vi "YKMW100 Measurement Single Analog Channel Data.vi"(0 "VISA session":refnum<visa-resource-name>, 1 "How to Get Data (F:Binary)":bool, 5 "Start Channel (001)":string="001", 9 "End Channel (001)":string="001", 11 "error in (no error)":errorcluster, 12 "Decimal Place List (no array)":i8[](array[numeric]) min=-1 max=4 step=1) -> (2 "Date Time":T1={"Year"=0, "Month"=1, "Day"=1, "Hour"=0, "Minute"=0, "Second"=0} {"Second" max=59 step=1; "Minute" max=59 step=1; "Hour" max=23 step=1; "Day" min=1 max=31 step=1; "Month" min=1 max=12 step=1; "Year" max=99 step=1}, 4 "dup VISA session":refnum<visa-resource-name>, 6 "Channel List":string[](array[string]), 8 "Data List":dbl[](array[numeric]) format="%.4f", 10 "Data Status List":T3(array[ring]), 13 "Alarm Status List":T2(array[cluster]), 14 "Decimal Place List":i8[](array[numeric]) min=-1 max=4 step=1, 15 "error out":errorcluster)   [LabVIEW 2009]
doc: "This VI gets the measurement data by ASCII or BINARY.\nWhen the data is formated by binary and the decimal place list is no array, this VI gets the unit and decimal point information by YKMW100 Unit Decimal Point.vi."
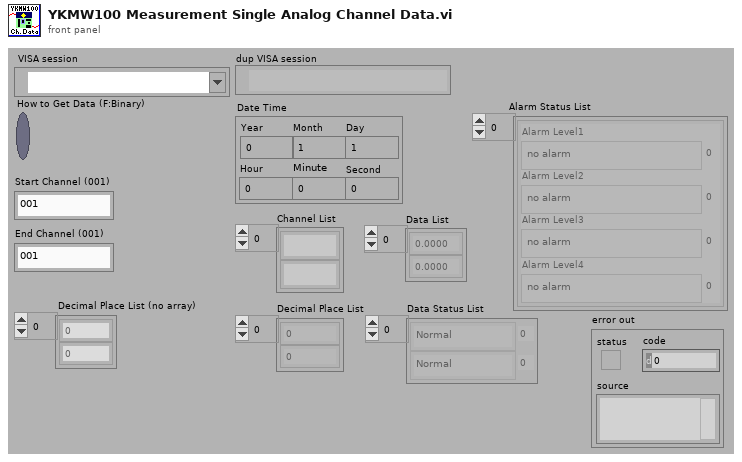
[diagram p1: front panel]
types:
  T1 = cluster{"Year":u8, "Month":u8, "Day":u8, "Hour":u8, "Minute":u8, "Second":u8}
  T2 = cluster{"Alarm Level1":enum8{"no alarm", "H (upper limit)", "L (lower Limit)", "h (defference upper limit)", "l (difference lower limit)", "R (upper limit on rate of change)", "r (lower limit on rate of change)"}, "Alarm Level2":enum8{"no alarm", "H (upper limit)", "L (lower Limit)", "h (defference upper limit)", "l (difference lower limit)", "R (upper limit on rate of change)", "r (lower limit on rate of change)"}, "Alarm Level3":enum8{"no alarm", "H (upper limit)", "L (lower Limit)", "h (defference upper limit)", "l (difference lower limit)", "R (upper limit on rate of change)", "r (lower limit on rate of change)"}, "Alarm Level4":enum8{"no alarm", "H (upper limit)", "L (lower Limit)", "h (defference upper limit)", "l (difference lower limit)", "R (upper limit on rate of change)", "r (lower limit on rate of change)"}}[]
  T3 = enum8{"Normal", "Differential Input", "Skip", "Over", "Error"}[]
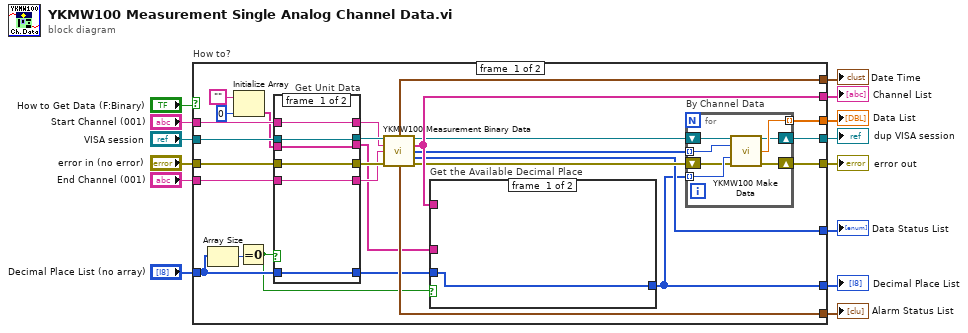
[diagram p0: block diagram]
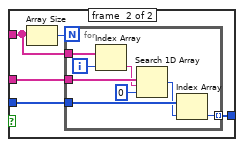
[diagram p2: hidden frame]
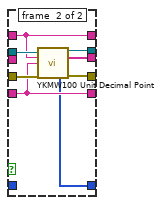
[diagram p3: hidden frame]
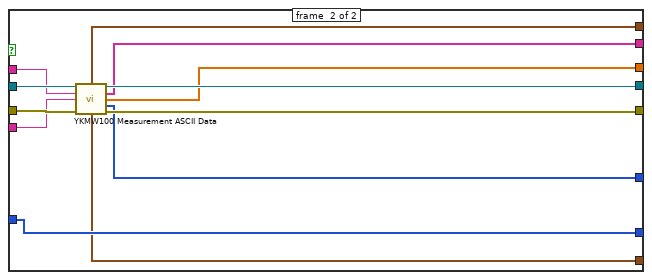
[diagram p4: hidden frame]
diagram:
  n1 = case "How to?" shown="False" "How to Get Data (F:Binary)" {
    tunnel: "VISA session" -> [w41 w87]
    tunnel: "error in (no error)" -> [w40 w86]
    tunnel: [w31 w82] -> w12
    tunnel: [w30 w81] -> w11
    tunnel: "End Channel (001)" -> [w38 w85]
    tunnel: "Start Channel (001)" -> [w39 w84]
    tunnel: "Decimal Place List (no array)" -> [w37 w88]
    tunnel: [w15 w88] -> w8
    tunnel: [w28 w83] -> w7
    tunnel: [w29 w78] -> w6
    tunnel: [w16 w79] -> w5
    tunnel: [w27 w80] -> w4
    tunnel: [w26 w77] -> w1
    frame #0 {
      n2 = Array Size(array=w37) -> (size(s)=w36:i32)
      n3 = Initialize Array("", 0) -> (w20:string[])
      n4 = Equal To 0?(x=w36) -> (x = 0?=w23:bool)
      n5 = case "Get Unit Data" shown="True" w23 {
        tunnel: w41 -> [w68 w76]
        tunnel: w40 -> [w67 w75]
        tunnel: w39 -> [w66 w72]
        tunnel: w38 -> [w65 w71]
        tunnel: [w67 w74] -> w34
        tunnel: [w68 w73] -> w35
        tunnel: [w66 w72] -> w33
        tunnel: [w65 w71] -> w32
        tunnel: [w64 w70] -> w24
        tunnel: w37 -> [w64 _]
        tunnel: [w63 w69] -> w25
        tunnel: w20 -> [w63 _]
        frame #0 {
        }
        frame #1 {
          n6 = call <instrlib>:"YKMW100 Unit Decimal Point.vi"("VISA session"=w76, "Start Channel (001)"=w72, "End Channel (001)"=w71, "error in (no error)"=w75) -> ("dup VISA session"=w73:refnum<visa-resource-name>, "Channel List"=w69:string[], "Decimal Place List"=w70:i8[], "error out"=w74:errorcluster)  [unwired: 6 in, 2 out]
        }
      }
      n7 = call <instrlib>:"YKMW100 Measurement Binary Data.vi"("VISA session"=w35, "Start Channel (001)"=w33, "End Channel (001)"=w32, "error in (no error)"=w34) -> ("Date Time"=w28:T1, "dup VISA session"=w19:refnum<visa-resource-name>, "Channel List"=w26:string[], "Data List"=w18:i32[], "Data Status List"=w16:T3, "Alarm Status List"=w27:T2, "error out"=w17:errorcluster)  [unwired: 5 in]
      n8 = case "Get the Available Decimal Place" shown="True" w23 {
        tunnel: w25 -> [_ w47]
        tunnel: w24 -> [w42 w46]
        tunnel: [w42 w45] -> w15
        tunnel: w26 -> [_ w43]
        frame #0 {
        }
        frame #1 {
          n9 = Array Size(array=w43) -> (size(s)=w44:i32)
          n10 = for {
            N: w44 -> [_]
            tunnel: w43 -> [w55]
            tunnel: w47 -> [w53]
            tunnel: w46 -> [w51]
            tunnel: [w49] -> w45 mode=indexing
            i -> [w54]
            n11 = Index Array(array=w55, index=w54) -> (element=w52:string)
            n12 = Search 1D Array(1D array=w53, element=w52, start index (0)=u8 0 ("開始指標（0）")) -> (index of element=w50:i32)
            n13 = Index Array(array=w51, index=w50) -> (element=w49:i8)
          }
        }
      }
      n14 = for "By Channel Data" {
        shift-right: [w60] -> w30
        shift-left: w17 -> [w61]
        tunnel: w18 -> [w58] mode=indexing
        tunnel: w15 -> [w62] mode=indexing
        tunnel: [w57] -> w29 mode=indexing
        shift-right: [w56] -> w31
        shift-left: w19 -> [w59]
        n15 = call <instrlib>:"YKMW100 Make Data.vi"("VISA session"=w59, "Measurement Data (0)"=w58, "Decimal Place (0)"=w62, "error in (no error)"=w61) -> ("dup VISA session"=w56:refnum<visa-resource-name>, "Data (0.0000)"=w57:dbl, "error out"=w60:errorcluster)  [unwired: 9 in]
      }
    }
    frame #1 {
      n16 = call <instrlib>:"YKMW100 Measurement ASCII Data.vi"("VISA session"=w87, "Start Channel (001)"=w84, "End Channel (001)"=w85, "error in (no error)"=w86) -> ("Date Time"=w83:T1, "dup VISA session"=w82:refnum<visa-resource-name>, "Channel List"=w77:string[], "Data List"=w78:dbl[], "Data Status List"=w79:T3, "Alarm Status List"=w80:T2, "error out"=w81:errorcluster)  [unwired: 4 in, 1 out]
    }
  }
  "error out" <- w11
  "dup VISA session" <- w12
  "Decimal Place List" <- w8
  "Data Status List" <- w5
  "Alarm Status List" <- w4
  "Date Time" <- w7
  "Data List" <- w6
  "Channel List" <- w1
